vi "reboot.vi"() -> ()   [LabVIEW 2016]
uses:
  dxl_x86_c.lvlib/dxl_x86_c.lvlib
panel:
  out "dynamixel_error":string
  out "dynamixel_comm_result":string
  in  "device_name":string="COM1"
  out "protocol_version":dbl=2.0
  out "port_num":i32
  in  "dynamixel_id":u8=1
  in  "baud_rate":i32=57600
  # "/*******************************************************************************\n* Copyright (c) 2016, ROBOTIS CO., LTD.\n* All rights reserved.\n*\n* Redistribution and use in source and binary forms, with or without\n* modification, are permitted provided that the following conditions are met:\n*\n* * Redistributions of source code must retain the above copyright notice, this\n*   list of conditions and the following disclaimer.\n*\n* * Redistributions in binary form must reproduce the above copyright notice,\n*   this list of conditions and the following disclaimer in the documentation\n*   and/or other materials provided with the distribution.\n*\n* * Neither the name of ROBOTIS nor the names of its\n*   contributors may be used to endorse or promote products derived from\n*   this software without specific prior written permission.\n*\n* THIS SOFTWARE IS PROVIDED BY THE COPYRIGHT HOLDERS AND CONTRIBUTORS \"AS IS\"\n* AND ANY EXPRESS OR IMPLIED WARRANTIES, INCLUDING, BUT NOT LIMITED TO, THE\n* IMPLIED WARRANTIES OF MERCHANTABILITY AND FITNESS FOR A PARTICULAR PURPOSE ARE\n* DISCLAIMED. IN NO EVENT SHALL THE COPYRIGHT HOLDER OR CONTRIBUTORS BE LIABLE\n* FOR ANY DIRECT, INDIRECT, INCIDENTAL, SPECIAL, EXEMPLARY, OR CONSEQUENTIAL\n* DAMAGES (INCLUDING, BUT NOT LIMITED TO, PROCUREMENT OF SUBSTITUTE GOODS OR\n* SERVICES; LOSS OF USE, DATA, OR PROFITS; OR BUSINESS INTERRUPTION) HOWEVER\n* CAUSED AND ON ANY THEORY OF LIABILITY, WHETHER IN CONTRACT, STRICT LIABILITY,\n* OR TORT (INCLUDING NEGLIGENCE OR OTHERWISE) ARISING IN ANY WAY OUT OF THE USE\n* OF THIS SOFTWARE, EVEN IF ADVISED OF THE POSSIBILITY OF SUCH DAMAGE.\n*******************************************************************************/\n\n/* Author: Ryu Woon Jung (Leon) */"
  # "Available Dynamixel model on this example : All models using Protocol 2.0\nThis example is designed for using a Dynamixel PRO 54-200, and an USB2DYNAMIXEL.\nTo use another Dynamixel model, such as X series, see their details in E-Manual(support.robotis.com) \n   and edit \"numeric control\"s seen left with \"Edit Text\" tool.\nBe sure that Dynamixel PRO properties are already set as %% ID : 1 / Baudnum : 1 (Baudrate : 57600)\n\n1. Run example by click above \"Run\" button (below \"Edit\" menu).\n2. The Dynamixel will reboot while Dynamixel LED is flickering"
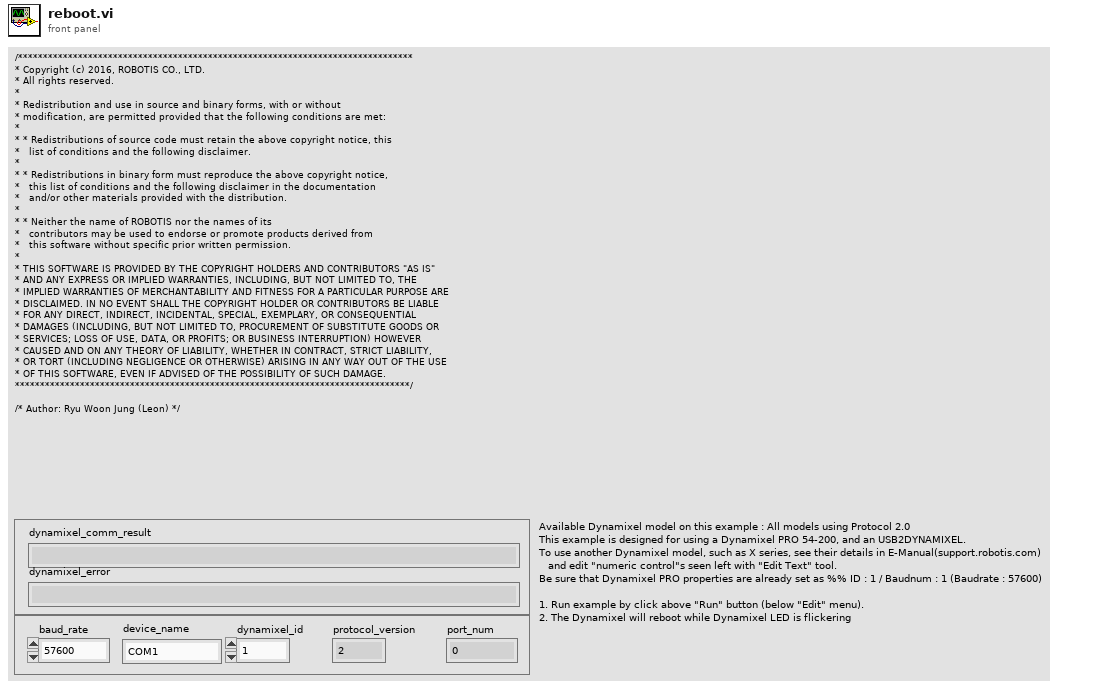
[diagram p1: front panel]
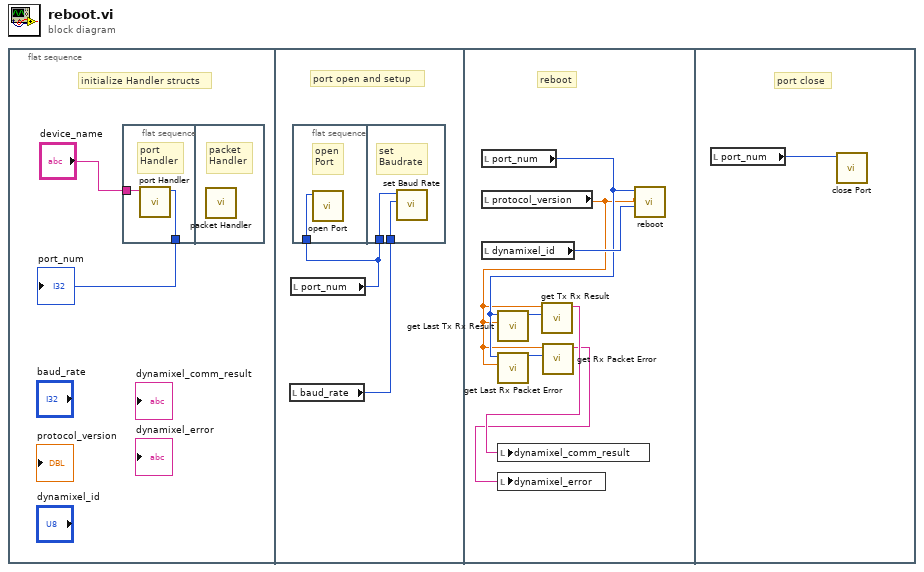
[diagram p0: block diagram]
diagram:
  n1 = flat-sequence {
    frame #0 {
      # "initialize Handler structs"
      n2 = flat-sequence {
        tunnel: [w4] -> w2
        tunnel: "device_name" -> [w3]
        frame #0 {
          # "port\nHandler"
          n3 = call "port Handler.vi"("port_name"=w3) -> ("function return"=w4:i32)  [unwired: 10 in]
        }
        frame #1 {
          # "packet\nHandler"
          n4 = call "packet Handler.vi"() -> ()  [unwired: 12 in]
        }
      }
      "port_num" <- w2
    }
    frame #1 {
      # "port open and setup"
      n5 = local read "baud_rate"() -> (w5:i32)
      n6 = local read "port_num"() -> (w6:i32)
      n7 = flat-sequence {
        tunnel: w6 -> [w7]
        tunnel: w6 -> [w9]
        tunnel: w5 -> [w8]
        frame #0 {
          # "open\nPort"
          n8 = call "open Port.vi"("port_num"=w7) -> ()  [unwired: 10 in, 1 out]
        }
        frame #1 {
          # "set\nBaudrate"
          n9 = call "set Baud Rate.vi"("baudrate"=w8, "port_num"=w9) -> ()  [unwired: 9 in, 1 out]
        }
      }
    }
    frame #2 {
      # "reboot"
      n10 = local read "port_num"() -> (w11:i32)
      n11 = local read "protocol_version"() -> (w10:dbl)
      n12 = local read "dynamixel_id"() -> (w16:u8)
      n13 = call "get Last Tx Rx Result.vi"("protocol_version"=w10, "port_num"=w11) -> ("function return"=w15:i32)  [unwired: 9 in]
      n14 = call "get Last Rx Packet Error.vi"("protocol_version"=w10, "port_num"=w11) -> ("function return"=w14:u8)  [unwired: 9 in]
      n15 = call "get Tx Rx Result.vi"("result"=w15, "protocol_version"=w10) -> ("function return"=w13:string)  [unwired: 9 in]
      n16 = local write "dynamixel_comm_result"(w13) -> ()
      n17 = call "get Rx Packet Error.vi"("error"=w14, "protocol_version"=w10) -> ("function return"=w12:string)  [unwired: 9 in]
      n18 = local write "dynamixel_error"(w12) -> ()
      n19 = call "reboot.vi"("id"=w16, "protocol_version"=w10, "port_num"=w11) -> ()  [unwired: 9 in]
    }
    frame #3 {
      # "port close"
      n20 = local read "port_num"() -> (w17:i32)
      n21 = call "close Port.vi"("port_num"=w17) -> ()  [unwired: 11 in]
    }
  }
